vi "TB-Load Calibration Log.vi"(0 "Cal Log":path) -> (4 "Log":string[][](array[string]), 6 "mean value":dbl)   [LabVIEW 2020]
uses:
  <vilib>/gmath/NI_Gmath.lvlib
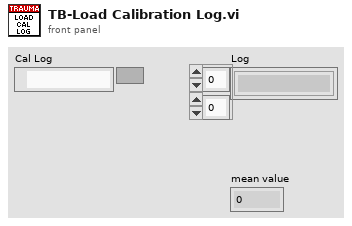
[diagram p1: front panel]
types:
  T1 = enum16{"arithmetic", "geometric", "harmonic", "trimmed", "median"}
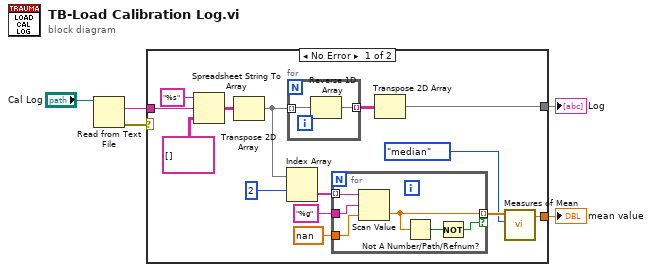
[diagram p0: block diagram]
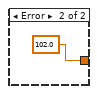
[diagram p2: hidden frame]
diagram:
  n1 = Read from Text File(file (use dialog)="Cal Log") -> (text=w3:string, error out=w2:errorcluster)  [unwired: 3 in, 2 out]
  n2 = case shown="No Error" w2 {
    tunnel: w3 -> [w19 _]
    tunnel: [w14 _] -> w4
    tunnel: [w6 102.0] -> w5
    frame No Error {
      n3 = Spreadsheet String To Array(format string="%s", spreadsheet string=w19, array type (2D Dbl)=string[][] []) -> (array=w16:string[][])  [unwired: 1 in]
      n4 = Transpose 2D Array(2D array=w16) -> (transposed array=w13:string[][])
      n5 = Index Array(array=w13, index (row)=2) -> (element=w11:string[])  [unwired: 1 in]
      n6 = for {
        tunnel: w13 -> [w27] mode=indexing
        tunnel: [w26] -> w15 mode=indexing
        n7 = Reverse 1D Array(array=w27) -> (reversed array=w26:string[])
      }
      n8 = for {
        tunnel: w11 -> [w25] mode=indexing
        tunnel: "%g" ("format string") -> [w24]
        tunnel: [w22] -> w8 mode=indexing if=w20
        tunnel: nan ("default (0 dbl)") -> [w23]
        n9 = Scan Value(string=w25, format string=w24, default (0 dbl)=w23) -> (value=w22:dbl)  [unwired: 1 out]
        n10 = Not A Number/Path/Refnum?(number/path/refnum=w22) -> (NaN/Path/Refnum?=w21:bool)
        n11 = Not(x=w21) -> (.not. x?=w20:bool)
      }
      n12 = Transpose 2D Array(2D array=w15) -> (transposed array=w14:string[][])
      n13 = call <vilib>:"Measures of Mean.vi"("type"=T1."median", "x array"=w8) -> ("mean value"=w6:dbl)  [unwired: 8 in, 1 out]
    }
    frame Error {
    }
  }
  "mean value" <- w5
  "Log" <- w4
